vi "Parse State Name from Menu Item Tag.vi"(8 "error in (no error)":errorcluster, 11 "Menu Item Tag Suffix in":string) -> (0 "error out":errorcluster, 2 "Action":string, 3 "State Name":string)   [LabVIEW 2013]
uses:
  <userlib>/_OpenG.lib/string/string.llb/Trim Whitespace (String)__ogtk.vi
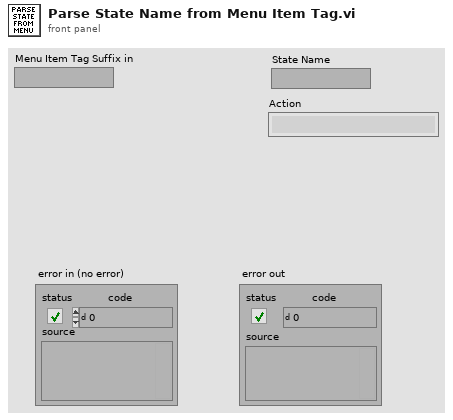
[diagram p1: front panel]
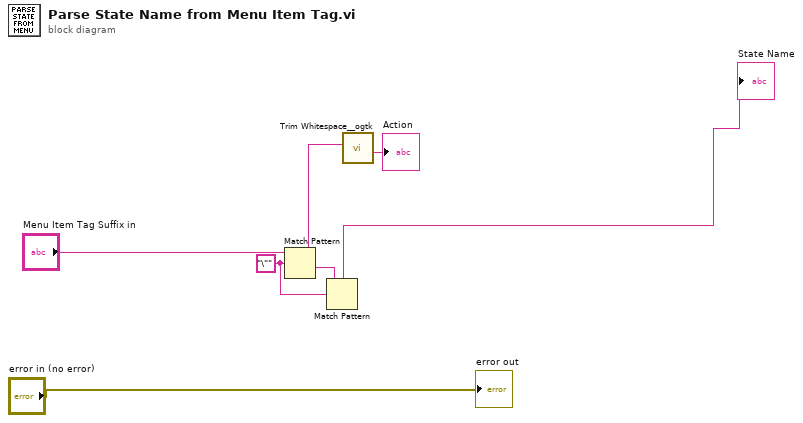
[diagram p0: block diagram]
diagram:
  w4 = "\"" ("regular expression")
  n1 = Match Pattern(string="Menu Item Tag Suffix in", regular expression=w4) -> (before substring=w2:string, after substring=w5:string)  [unwired: 1 in, 2 out]
  n2 = Match Pattern(string=w5, regular expression=w4) -> (before substring=→"State Name":string)  [unwired: 1 in, 3 out]
  n3 = call-poly <userlib>:"Trim Whitespace__ogtk.vi"("String in"=w2) -> ("String out"=→"Action":string)  [unwired: 6 in]
  "error out" <- "error in (no error)"
